vi "Reformat.vi"(4 "Disable LabVIEW Extensions":bool, 5 "Format empty string as null":bool, 6 "Pretty Print Levels":i32, 7 "Alphabetically Sort Objects":bool, 8 "error in (no error)":errorcluster, 10 "Offset":i32, 11 "JSON":string) -> (0 "error out":errorcluster, 1 "Offset past":i32 caption="Offset past Value", 2 "Rest of Input String":string, 3 "<JSON>":string caption="<JSON>First JSON Value")   [LabVIEW 2019, in "JSONtext.lvlib"]
doc: "Reformat a JSON Value, either packed with all unneeded whitespace removed, or \"pretty printed\" with extra whitespace and new lines to make the JSON more human readable. This will also serve to validate the JSON.\n\n\"Pretty Print Levels\" is the number of deeper levels at which to apply pretty print. Use a high number to apply at all levels, and use zero to indicate no pretty print."
uses:
  JSONtext.lvlib
  Parsing/Advance past Line Ending.vi
  String Subset.vi
  <vilib>/Utility/error.llb/Error Cluster From Error Code.vi
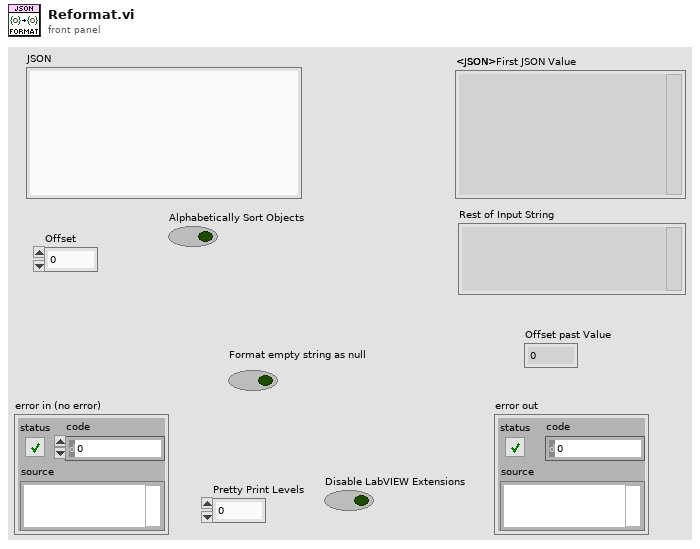
[diagram p1: front panel]
types:
  T1 = typedef "JSONtext.lvlib/Parsing State.ctl" = enum16{"Parser Error", "Object", "Array", "String", "Number/Other", "Leading Whitespace", "Object end", "Array end", "Value end"}
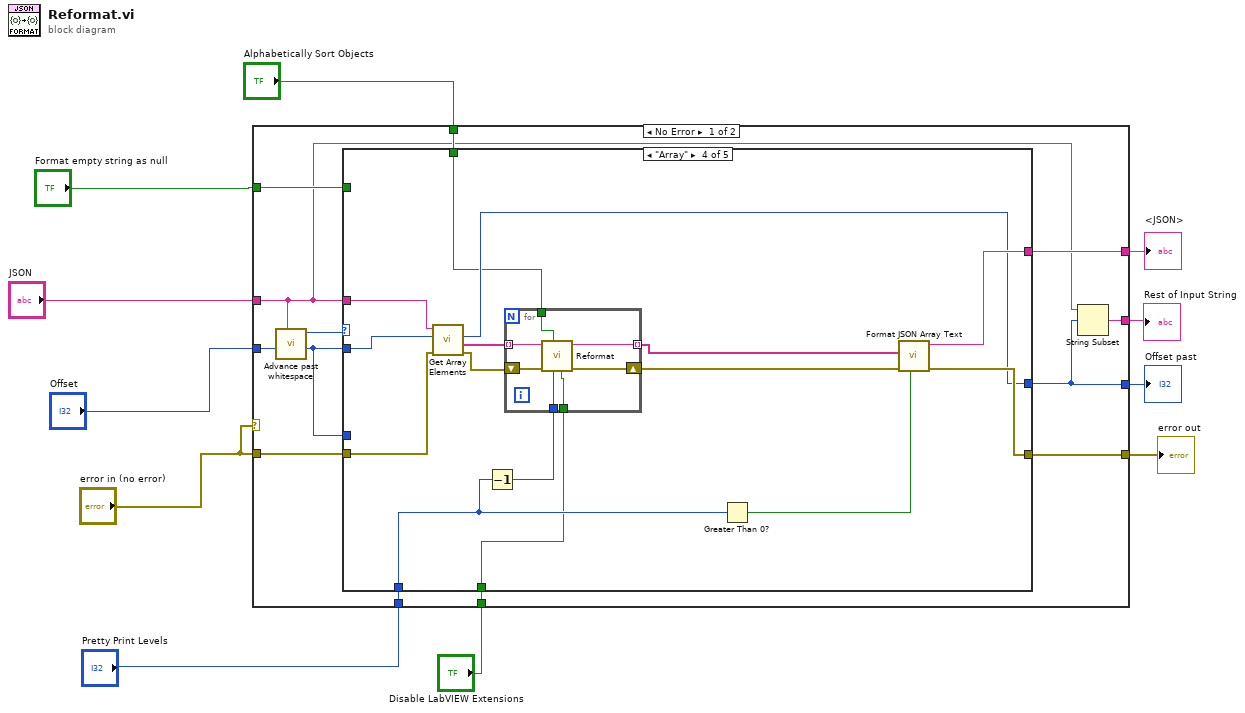
[diagram p0: block diagram]
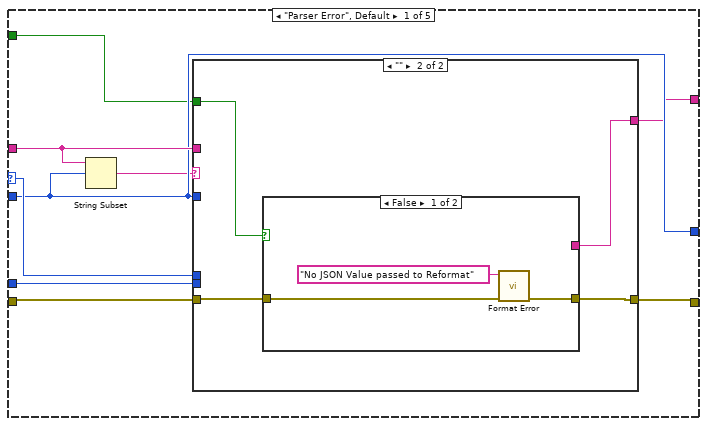
[diagram p2: hidden frame]
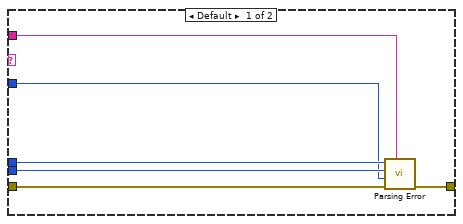
[diagram p3: hidden frame]
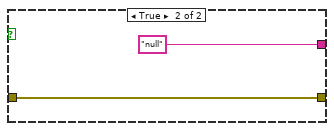
[diagram p4: hidden frame]
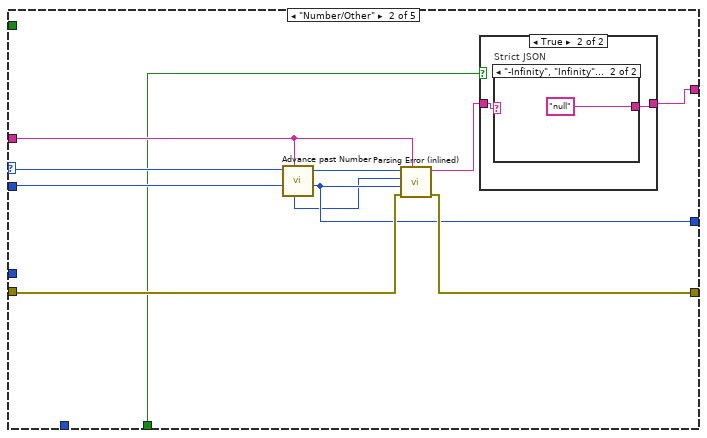
[diagram p5: hidden frame]
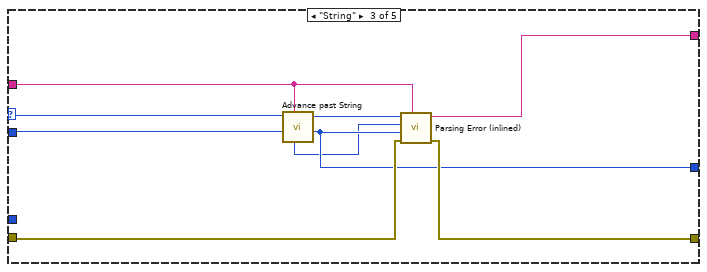
[diagram p8: hidden frame]
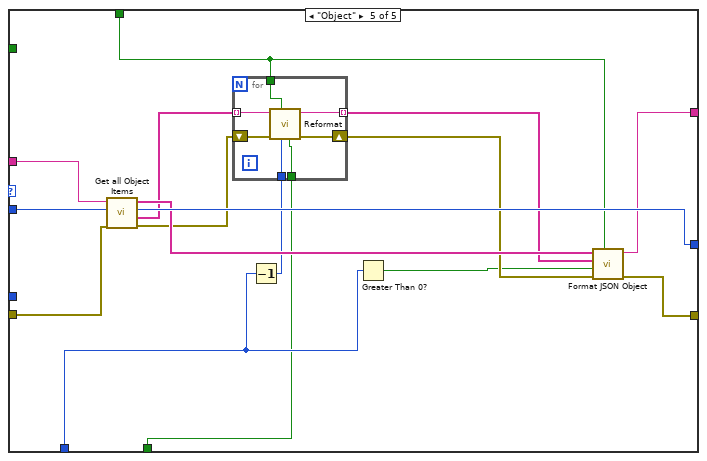
[diagram p9: hidden frame]
diagram:
  n1 = case shown="No Error" "error in (no error)" {
    tunnel: "JSON" -> [w13 w120]
    tunnel: "Offset" -> [w23 w121]
    tunnel: [w22 w119] -> w9
    tunnel: "error in (no error)" -> [w21 w119]
    tunnel: "Pretty Print Levels" -> [w19 _]
    tunnel: [w18 _] -> w7
    tunnel: [w17 w121] -> w6
    tunnel: [w16 w120] -> w5
    tunnel: "Alphabetically Sort Objects" -> [w15 _]
    tunnel: "Format empty string as null" -> [w14 _]
    tunnel: "Disable LabVIEW Extensions" -> [w12 _]
    frame No Error {
      n2 = call "Advance past whitespace.vi"("JSON"=w13, "Offset"=w23) -> ("Offset of first non-whitespace"=w20:i32, "Parser State"=w24:T1)  [unwired: 7 in, 1 out]
      n3 = case shown="\"Array\"" w24 {
        selector: w24 -> [w31 w59 w73 _ _]
        tunnel: w13 -> [w29 w52 w66 w88 w108]
        tunnel: w20 -> [w28 w58 w72 w87 w111]
        tunnel: [w28 w55 w69 w81 w110] -> w17
        tunnel: [w26 w51 w65 w85 w107] -> w18
        tunnel: [w33 w56 w70 w83 w102] -> w22
        tunnel: w21 -> [w32 w57 w71 w82 w101]
        tunnel: w20 -> [w30 _ _ _ _]
        tunnel: w19 -> [_ _ _ w78 w99]
        tunnel: w15 -> [_ _ _ w75 w97]
        tunnel: w14 -> [w25 _ _ _ _]
        tunnel: w12 -> [_ w49 _ w74 w96]
        frame "Parser Error", Default {
          n4 = String Subset(string=w29, offset (0)=w28) -> (substring=w27:string)  [unwired: 1 in]
          n5 = case shown="\"\"" w27 {
            tunnel: [w39 w42] -> w33
            tunnel: w32 -> [w38 w43]
            tunnel: w31 -> [w37 _]
            tunnel: w30 -> [w36 _]
            tunnel: w29 -> [w35 _]
            tunnel: w28 -> [w34 _]
            tunnel: [_ w40] -> w26
            tunnel: w25 -> [_ w41]
            frame Default {
              n6 = call "Parsing Error.vi"("JSON"=w35, "error in (no error)"=w38, "Offset past match"=w34, "Value start"=w36, "State"=w37) -> ("error out"=w39:errorcluster)  [unwired: 6 in]
            }
            frame "" {
              n7 = case shown="False" w41 {
                tunnel: w43 -> [w46 w48]
                tunnel: [w45 w48] -> w42
                tunnel: [_ "null"] -> w40
                frame False {
                  n8 = call "Format Error.vi"("error in (no error)"=w46, "error message"="No JSON Value passed to Reformat") -> ("error out"=w45:errorcluster)  [unwired: 9 in]
                }
                frame True {
                }
              }
            }
          }
        }
        frame "Number/Other" {
          n9 = call "Advance past Number.vi"("JSON"=w52, "Offset (0)"=w58, "Parser State in"=w59) -> ("Offset past match"=w55:i32, "Parser State"=w53:T1, "Value start out"=w54:i32)  [unwired: 5 in, 1 out]
          n10 = call "Parsing Error (inlined).vi"("JSON"=w52, "error in (no error)"=w57, "Offset past match"=w55, "Value start"=w54, "State"=w53) -> ("error out"=w56:errorcluster, "Value (if no error)"=w50:string)  [unwired: 5 in]
          n11 = case shown="True" w49 {
            tunnel: w50 -> [w60 w62]
            tunnel: [w60 w61] -> w51
            frame False {
            }
            frame True {
              n12 = case "Strict JSON" shown="\"-Infinity\", \"Infinity\", \"NaN\"" w62 {
                selector: w62 -> [w63 _]
                tunnel: [w63 "null"] -> w61
                frame Default {
                }
                frame "-Infinity", "Infinity", "NaN" {
                }
              }
            }
          }
        }
        frame "String" {
          n13 = call "Advance past String.vi"("JSON"=w66, "Offset"=w72, "State in"=w73) -> ("Offset past match"=w69:i32, "State"=w67:T1, "Value start out"=w68:i32)  [unwired: 6 in]
          n14 = call "Parsing Error (inlined).vi"("JSON"=w66, "error in (no error)"=w71, "Offset past match"=w69, "Value start"=w68, "State"=w67) -> ("error out"=w70:errorcluster, "Value (if no error)"=w65:string)  [unwired: 5 in]
        }
        frame "Array" {
          n15 = call "Get Array Elements.vi"("error in (no error)"=w82, "Offset"=w87, "JSON"=w88) -> ("error out"=w84:errorcluster, "<JSON>"=w86:string[], "Offset past"=w81:i32)  [unwired: 6 in]
          n16 = Decrement(x=w78) -> (x-1=w77:i32)
          n17 = for {
            tunnel: w86 -> [w95] mode=indexing
            tunnel: [w94] -> w80 mode=indexing
            shift-right: [w92] -> w79
            shift-left: w84 -> [w93]
            tunnel: w77 -> [w91]
            tunnel: w75 -> [w90]
            tunnel: w74 -> [w89]
            n18 = call "Reformat.vi"("Disable LabVIEW Extensions"=w89, "Pretty Print Levels"=w91, "Alphabetically Sort Objects"=w90, "error in (no error)"=w93, "JSON"=w95) -> ("error out"=w92:errorcluster, "<JSON>"=w94:string)  [unwired: 3 in, 2 out]
          }
          n19 = Greater Than 0?(x=w78) -> (x > 0?=w76:bool)
          n20 = call "Format JSON Array Text.vi"("Pretty Print?"=w76, "error in (no error)"=w79, "Array of JSON Text"=w80) -> ("error out"=w83:errorcluster, "<JSON>"=w85:string)  [unwired: 7 in]
        }
        frame "Object" {
          n21 = call "Get all Object Items.vi"("error in (no error)"=w101, "Offset"=w111, "JSON"=w108) -> ("error out"=w104:errorcluster, "<JSON>"=w106:string[], "Offset past"=w110:i32, "Item Names"=w109:string[])  [unwired: 5 in]
          n22 = Decrement(x=w99) -> (x-1=w98:i32)
          n23 = for {
            tunnel: w106 -> [w118] mode=indexing
            tunnel: [w117] -> w105 mode=indexing
            shift-right: [w115] -> w103
            shift-left: w104 -> [w116]
            tunnel: w98 -> [w114]
            tunnel: w97 -> [w113]
            tunnel: w96 -> [w112]
            n24 = call "Reformat.vi"("Disable LabVIEW Extensions"=w112, "Pretty Print Levels"=w114, "Alphabetically Sort Objects"=w113, "error in (no error)"=w116, "JSON"=w118) -> ("error out"=w115:errorcluster, "<JSON>"=w117:string)  [unwired: 3 in, 2 out]
          }
          n25 = Greater Than 0?(x=w99) -> (x > 0?=w100:bool)
          n26 = call "Format JSON Object.vi"("Alphabetical Sort"=w97, "error in (no error)"=w103, "Pretty Print?"=w100, "JSON elements"=w105, "Names"=w109) -> ("error out"=w102:errorcluster, "JSON Object Text out"=w107:string)  [unwired: 5 in]
        }
      }
      n27 = String Subset(string=w13, offset (0)=w17) -> (substring=w16:string)  [unwired: 1 in]
    }
    frame Error {
    }
  }
  "Offset past" <- w6
  "<JSON>" <- w7
  "error out" <- w9
  "Rest of Input String" <- w5
